vi "Write Char Data to S2P.vi"(0 "VISA resource name":refnum<visa-resource-name>, 1 "S2P File Path In":path, 5 "ACM Path":T1, 11 "error in (no error)":errorcluster) -> (3 "S2P File Path Out":path, 4 "VISA resource name out":refnum<visa-resource-name>, 15 "error out":errorcluster)   [LabVIEW 2023, in "ACM Visa Driver.lvlib"]
uses:
  ACM Visa Driver.lvlib
  API/Controls/ACM Paths.ctl
  HFNetworkAnalysis/Controls/SnPDataType.ctl
  API/Controls/ACM S-Parameters.ctl
  HFNetworkAnalysis/NI_HFNetworkAnalysis.lvlib
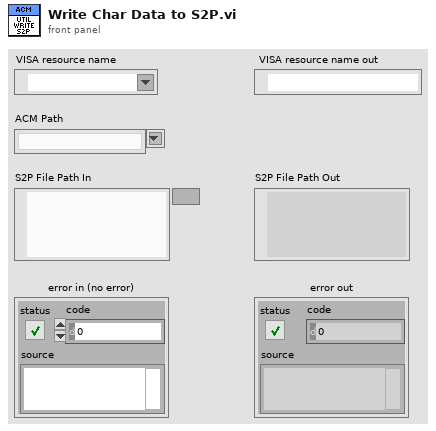
[diagram p1: front panel]
types:
  T1 = typedef "ACM Visa Driver.lvlib/ACM Paths.ctl" = string
  T2 = typedef "ACM Visa Driver.lvlib/ACM S-Parameters.ctl" = string
  T3 = typedef "NI_HFNetworkAnalysis.lvlib/SnPDataType.ctl" = enum16{"DB", "MA", "RI"}
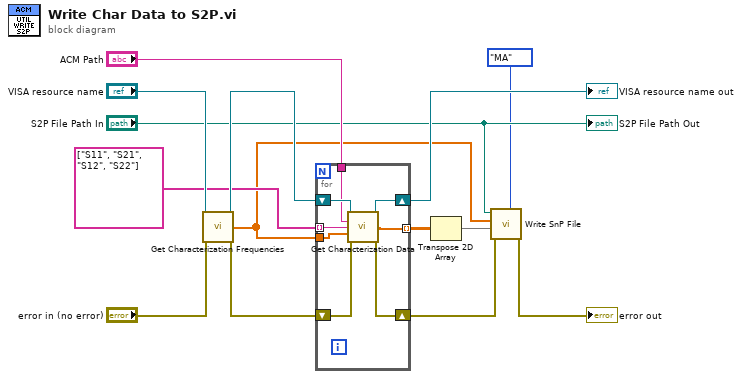
[diagram p0: block diagram]
diagram:
  n1 = call "Get Characterization Frequencies.vi"("VISA resource name"="VISA resource name", "error in (no error)"="error in (no error)") -> ("VISA resource name out"=w14:refnum<visa-resource-name>, "S-Par Characterization Frequencies"=w1:dbl[], "error out"=w13:errorcluster)  [unwired: 11 in]
  n2 = for {
    tunnel: "ACM Path" -> [w19]
    tunnel: T2[] ["S11", "S21", "S12", "S22"] ("Array") -> [w18] mode=indexing
    shift-right: [w17] -> w6
    shift-left: w14 -> [w22]
    shift-right: [w20] -> w10
    shift-left: w13 -> [w21]
    tunnel: [w16] -> w3 mode=indexing
    tunnel: w1 -> [w15]
    n3 = call "Get Characterization Data.vi"("VISA resource name"=w22, "ACM Path"=w19, "S-Parameter"=w18, "Characterization Frequencies (for Temp Co)"=w15, "error in (no error)"=w21) -> ("VISA resource name out"=w17:refnum<visa-resource-name>, "S-Par Characterization Data"=w16:cdb[], "error out"=w20:errorcluster)  [unwired: 8 in]
  }
  "VISA resource name out" <- w6
  n4 = Transpose 2D Array(2D array=w3) -> (transposed array=w2:cdb[][])
  n5 = call "Write SnP File.vi"("OutputDataType"=SnPDataType."MA", "error in (no error)"=w10, "S-parameters"=w2, "Frequencies (Hz)"=w1, "SnP File Path"="S2P File Path In") -> ("error out"=→"error out":errorcluster)  [unwired: 6 in]
  "S2P File Path Out" <- "S2P File Path In"
